vi "global.vi"() -> ()   [LabVIEW 2018]
panel:
  in  "串口列表":string[](array[string])
  in  "测量距离":dbl
  in  "频率变化次数":dbl
  in  "电机移动次数":dbl
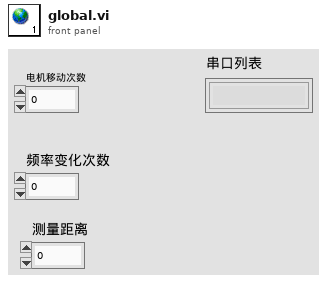
[diagram p1: front panel]
diagram:
